vi "Construct (Scalar).vi"(8 "Error in (no error)":errorcluster, 10 "Priority":T1 items=["EMERGENCY", "ALERT", "CRITICAL", "ERROR", "WARNING", "NOTICE", "INFO", "DEBUG"], 11 "LogFilterPriority in":refnum<class "LogFilterPriority.lvclass">) -> (0 "Error out":errorcluster, 3 "LogFilterPriority out":refnum<class "LogFilterPriority.lvclass">)   [LabVIEW 2011, in "LogFilterPriority.lvclass"]
uses:
  LogFilterPriority.lvclass
  Log/PrioritiesRing.ctl
  Log/Log.lvclass
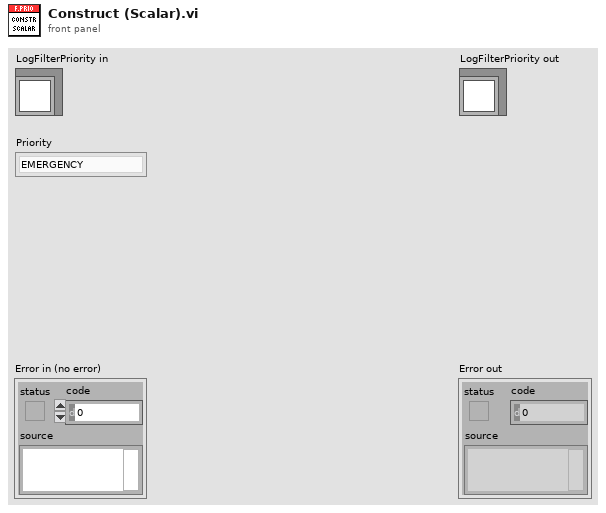
[diagram p1: front panel]
types:
  T1 = typedef "Log.lvclass/PrioritiesRing.ctl" = u32
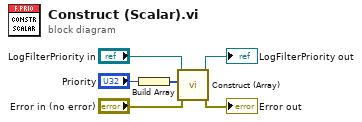
[diagram p0: block diagram]
diagram:
  n1 = Build Array("Priority") -> (w5:T1[])
  n2 = call "Construct (Array).vi"("Error in (no error)"="Error in (no error)", "Priorities"=w5, "LogFilterPriority in"="LogFilterPriority in") -> ("Error out"=→"Error out":errorcluster, "LogFilterPriority out"=→"LogFilterPriority out":refnum<class "LogFilterPriority.lvclass">)  [unwired: 7 in]
